vi "CRYPull Data From ProjectViewCluster Array.vi"() -> (2 "Is Remain ?":bool, 3 "ProjectViewCluster Out":T1)   [LabVIEW 2013]
uses:
  CRYSystem/Typedef Control/CRYProjectViewCluster.ctl
  CRYProject Editor Global.vi
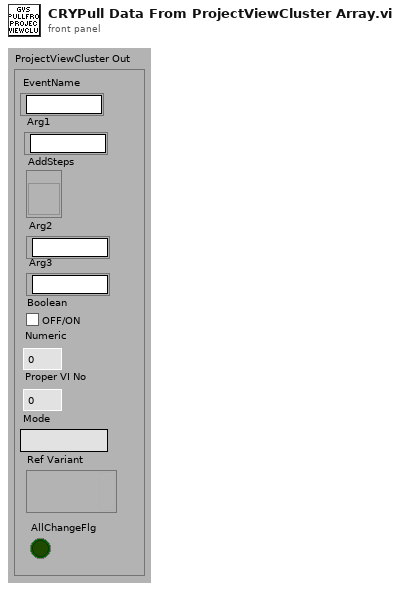
[diagram p1: front panel]
types:
  T1 = typedef "CRYProjectViewCluster.ctl" = cluster{"EventName":string, "Arg1":string, "Numeric":i32, "Proper VI No":i32, "AddSteps ":refnum<vi>, "Arg2":string, "Arg3":string, "Boolean":bool, "Mode":string, "Ref Variant":variant, "AllChangeFlg":bool}
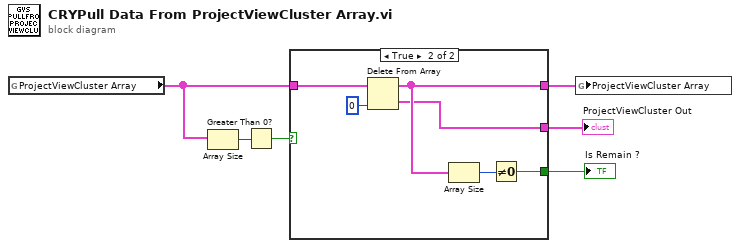
[diagram p0: block diagram]
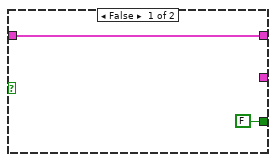
[diagram p2: hidden frame]
diagram:
  n1 = global read "CRYProject Editor Global.vi" "ProjectViewCluster Array"() -> (w3:T1[])
  n2 = Array Size(array=w3) -> (size(s)=w2:i32)
  n3 = Greater Than 0?(x=w2) -> (x > 0?=w1:bool)
  n4 = case shown="True" w1 {
    tunnel: w3 -> [w8 w14]
    tunnel: [w8 w12] -> w6
    tunnel: [FALSE w10] -> w5
    tunnel: [_ w9] -> w4
    frame False {
    }
    frame True {
      n5 = Delete From Array(array=w14, index=0) -> (deleted portion=w9:T1, array with subset deleted=w12:T1[])  [unwired: 1 in]
      n6 = Array Size(array=w12) -> (size(s)=w11:i32)
      n7 = Not Equal To 0?(x=w11) -> (x != 0?=w10:bool)
    }
  }
  "Is Remain ?" <- w5
  "ProjectViewCluster Out" <- w4
  n8 = global write "CRYProject Editor Global.vi" "ProjectViewCluster Array"(w6) -> ()
